vi "find splitting-fit lorentzian method.vi"(9 "E":dbl[][](graph)=array801x69[55269 elements], 10 "Y Scale":T2={"Offset"=-90000.0, "Multiplier"=2608.695652173913}, 11 "X Scale":T2={"Offset"=-0.09, "Multiplier"=8.5e-05}) -> (3 "XY Graph 4":cluster{dbl[], dbl[]}[](graph)=[{[-0.06773, -0.06773, -0.06824, -0.068325, -0.06841, -0.06841, -0.068325, -0.06806999999999999, -0.06773, -0.06773, -0.06773, -0.06773, -0.067645, -0.06738999999999999, -0.06722, -0.06705, -0.06670999999999999, -0.06637, -0.0662, -0.06602999999999999, -0.065775, -0.06552, -0.06534999999999999, -0.06517999999999999, -0.06509499999999999, -0.06484, -0.064585, -0.06416, -0.06841, -0.068665, -0.068835, -0.069005, -0.069005, -0.06909, -0.06909, -0.06917499999999999, -0.06925999999999999, -0.06917499999999999, -0.06917499999999999, -0.06909, -0.06909, -0.069005, -0.069005, -0.06909, -0.06909, -0.06892, -0.06874999999999999, -0.06874999999999999, -0.06874999999999999, -0.06773, -0.067475, -0.067645, -0.067645, -0.067645, -0.067645, -0.067475, -0.067475, -0.067475, -0.06738999999999999, -0.06756, -0.067475, -0.06738999999999999, -0.06738999999999999, -0.06738999999999999, -0.06722, -0.066965, -0.06670999999999999, -0.06645499999999999, -0.066115, -0.065945, -0.065605, -0.06534999999999999, -0.06517999999999999, -0.064925, -0.06466999999999999, -0.064245, -0.06398999999999999, -0.06381999999999999, -0.06390499999999999, -0.06433, -0.06398999999999999, -0.06398999999999999, -0.06841, -0.06858, -0.068835, -0.06892, -0.069005, -0.069005, -0.06909, -0.06909, -0.06909, -0.06917499999999999, -0.06925999999999999, -0.06925999999999999, -0.06942999999999999, -0.06934499999999999, -0.06934499999999999, -0.06942999999999999], [-1304.0, -1304.3478260869597, 1304.3478260869597, 3913.0434782608645, 6521.739130434784, 9130.434782608689, 11739.130434782608, 14347.826086956513, 16956.521739130432, 19565.21739130435, 22173.913043478256, 24782.608695652176, 27391.30434782608, 30000.0, 32608.695652173905, 35217.391304347824, 37826.08695652174, 40434.78260869565, 43043.47826086957, 45652.17391304349, 48260.86956521738, 50869.5652173913, 53478.260869565216, 56086.956521739135, 58695.652173913055, 61304.347826086945, 63913.043478260865, 66521.73913043478, 37826.08695652174, 40434.78260869565, 43043.47826086957, 45652.17391304349, 48260.86956521738, 50869.5652173913, 53478.260869565216, 56086.956521739135, 58695.652173913055, 61304.347826086945, 63913.043478260865, 66521.73913043478, 69130.4347826087, 71739.1304347826, 71739.1304347826, 74347.82608695651, 76956.52173913043, 79565.21739130435, 82173.91304347827, 84782.60869565216, 87391.30434782608, -1304.0, -3913.0434782608645, -9130.434782608703, -11739.130434782608, -14347.826086956527, -16956.521739130432, -19565.21739130435, -22173.913043478256, -24782.608695652176, -27391.304347826088, -30000.0, -32608.695652173912, -35217.391304347824, -37826.08695652174, -40434.782608695656, -43043.47826086957, -45652.17391304348, -48260.86956521739, -50869.565217391304, -53478.260869565216, -56086.95652173913, -58695.65217391304, -61304.34782608696, -63913.04347826087, -66521.73913043478, -69130.4347826087, -71739.13043478261, -74347.82608695653, -76956.52173913043, -79565.21739130435, -82173.91304347826, -84782.60869565218, -84782.60869565218, -50869.565217391304, -53478.260869565216, -56086.95652173913, -58695.65217391304, -61304.34782608696, -63913.04347826087, -66521.73913043478, -69130.4347826087, -71739.13043478261, -74347.82608695653, -76956.52173913043, -79565.21739130435, -82173.91304347826, -84782.60869565218, -84782.60869565218, -87391.30434782608]}])   [LabVIEW 2013]
uses:
  <vilib>/Utility/miscctls.llb/LVOffsetAndMultiplierTypeDef.ctl
  <vilib>/Analysis/baseanly.llb/Mean (DBL).vi
  <vilib>/Analysis/NI_AAL_SigProc.lvlib
  <vilib>/Analysis/NI_AALBase.lvlib
panel:
  out "size(s)":i32=1
  in  "Tab Control":T1(tab)
  out "E 2":dbl[][](graph)
  in  "OK Button":bool
  out "Peak Detector":cluster{"X":dbl, "Y":dbl}[](graph)=[{"X"=-0.07546499999999999, "Y"=-90000.0}, {"X"=-0.06398999999999999, "Y"=-90000.0}, {"X"=-0.07690999999999999, "Y"=-87391.30434782608}, {"X"=-0.06942999999999999, "Y"=-87391.30434782608}, {"X"=-0.076995, "Y"=-84782.60869565218}, {"X"=-0.06934499999999999, "Y"=-84782.60869565218}, {"X"=-0.06398999999999999, "Y"=-84782.60869565218}, {"X"=-0.077165, "Y"=-82173.91304347826}, {"X"=-0.06942999999999999, "Y"=-82173.91304347826}, {"X"=-0.06433, "Y"=-82173.91304347826}, {"X"=-0.07708, "Y"=-79565.21739130435}, {"X"=-0.06925999999999999, "Y"=-79565.21739130435}, {"X"=-0.06390499999999999, "Y"=-79565.21739130435}, {"X"=-0.07725, "Y"=-76956.52173913043}, {"X"=-0.06925999999999999, "Y"=-76956.52173913043}, {"X"=-0.06381999999999999, "Y"=-76956.52173913043}, {"X"=-0.07741999999999999, "Y"=-74347.82608695653}, {"X"=-0.06917499999999999, "Y"=-74347.82608695653}, {"X"=-0.06398999999999999, "Y"=-74347.82608695653}, {"X"=-0.07750499999999999, "Y"=-71739.13043478261}, {"X"=-0.06909, "Y"=-71739.13043478261}, {"X"=-0.064245, "Y"=-71739.13043478261}, {"X"=-0.06909, "Y"=-69130.4347826087}, {"X"=-0.06466999999999999, "Y"=-69130.4347826087}, {"X"=-0.06909, "Y"=-66521.73913043478}, {"X"=-0.064925, "Y"=-66521.73913043478}, {"X"=-0.069005, "Y"=-63913.04347826087}, {"X"=-0.06517999999999999, "Y"=-63913.04347826087}, {"X"=-0.069005, "Y"=-61304.34782608696}, {"X"=-0.06534999999999999, "Y"=-61304.34782608696}, {"X"=-0.06892, "Y"=-58695.65217391304}, {"X"=-0.065605, "Y"=-58695.65217391304}, {"X"=-0.068835, "Y"=-56086.95652173913}, {"X"=-0.065945, "Y"=-56086.95652173913}, {"X"=-0.06858, "Y"=-53478.260869565216}, {"X"=-0.066115, "Y"=-53478.260869565216}, {"X"=-0.06841, "Y"=-50869.565217391304}, {"X"=-0.06645499999999999, "Y"=-50869.565217391304}, {"X"=-0.06670999999999999, "Y"=-48260.86956521739}, {"X"=-0.066965, "Y"=-45652.17391304348}, {"X"=-0.06722, "Y"=-43043.47826086957}, {"X"=-0.06738999999999999, "Y"=-40434.782608695656}, {"X"=-0.06373499999999999, "Y"=-40434.782608695656}, {"X"=-0.06738999999999999, "Y"=-37826.08695652174}, {"X"=-0.06330999999999999, "Y"=-37826.08695652174}, {"X"=-0.06738999999999999, "Y"=-35217.391304347824}, {"X"=-0.06330999999999999, "Y"=-35217.391304347824}, {"X"=-0.067475, "Y"=-32608.695652173912}, {"X"=-0.06330999999999999, "Y"=-32608.695652173912}, {"X"=-0.06756, "Y"=-30000.0}, {"X"=-0.063055, "Y"=-30000.0}, {"X"=-0.06738999999999999, "Y"=-27391.304347826088}, {"X"=-0.067475, "Y"=-24782.608695652176}, {"X"=-0.067475, "Y"=-22173.913043478256}, {"X"=-0.067475, "Y"=-19565.21739130435}, {"X"=-0.067645, "Y"=-16956.521739130432}, {"X"=-0.067645, "Y"=-14347.826086956527}, {"X"=-0.067645, "Y"=-11739.130434782608}, {"X"=-0.067645, "Y"=-9130.434782608703}, {"X"=-0.067475, "Y"=-3913.0434782608645}, {"X"=-0.06773, "Y"=-1304.3478260869597}, {"X"=-0.06824, "Y"=1304.3478260869597}, {"X"=-0.068325, "Y"=3913.0434782608645}, {"X"=-0.06841, "Y"=6521.739130434784}, {"X"=-0.06841, "Y"=9130.434782608689}, {"X"=-0.068325, "Y"=11739.130434782608}, {"X"=-0.06806999999999999, "Y"=14347.826086956513}, {"X"=-0.06773, "Y"=16956.521739130432}, {"X"=-0.06773, "Y"=19565.21739130435}, {"X"=-0.06773, "Y"=22173.913043478256}, {"X"=-0.06365, "Y"=22173.913043478256}, {"X"=-0.06773, "Y"=24782.608695652176}, {"X"=-0.06381999999999999, "Y"=24782.608695652176}, {"X"=-0.067645, "Y"=27391.30434782608}, {"X"=-0.06390499999999999, "Y"=27391.30434782608}, {"X"=-0.06738999999999999, "Y"=30000.0}, {"X"=-0.06722, "Y"=32608.695652173905}, {"X"=-0.06705, "Y"=35217.391304347824}, {"X"=-0.06841, "Y"=37826.08695652174}, {"X"=-0.06670999999999999, "Y"=37826.08695652174}, {"X"=-0.068665, "Y"=40434.78260869565}, {"X"=-0.06637, "Y"=40434.78260869565}, {"X"=-0.068835, "Y"=43043.47826086957}, {"X"=-0.0662, "Y"=43043.47826086957}, {"X"=-0.069005, "Y"=45652.17391304349}, {"X"=-0.06602999999999999, "Y"=45652.17391304349}, {"X"=-0.069005, "Y"=48260.86956521738}, {"X"=-0.065775, "Y"=48260.86956521738}, {"X"=-0.06909, "Y"=50869.5652173913}, {"X"=-0.06552, "Y"=50869.5652173913}, {"X"=-0.06909, "Y"=53478.260869565216}, {"X"=-0.06534999999999999, "Y"=53478.260869565216}, {"X"=-0.06917499999999999, "Y"=56086.956521739135}, {"X"=-0.06517999999999999, "Y"=56086.956521739135}, {"X"=-0.06925999999999999, "Y"=58695.652173913055}, {"X"=-0.06509499999999999, "Y"=58695.652173913055}, {"X"=-0.06917499999999999, "Y"=61304.347826086945}, {"X"=-0.06484, "Y"=61304.347826086945}, {"X"=-0.07750499999999999, "Y"=63913.043478260865}, {"X"=-0.06917499999999999, "Y"=63913.043478260865}, {"X"=-0.064585, "Y"=63913.043478260865}, {"X"=-0.077335, "Y"=66521.73913043478}, {"X"=-0.06909, "Y"=66521.73913043478}, {"X"=-0.06416, "Y"=66521.73913043478}, {"X"=-0.07725, "Y"=69130.4347826087}, {"X"=-0.06909, "Y"=69130.4347826087}, {"X"=-0.06390499999999999, "Y"=69130.4347826087}, {"X"=-0.07708, "Y"=71739.1304347826}, {"X"=-0.069005, "Y"=71739.1304347826}, {"X"=-0.06365, "Y"=71739.1304347826}, {"X"=-0.076995, "Y"=74347.82608695651}, {"X"=-0.06909, "Y"=74347.82608695651}, {"X"=-0.06365, "Y"=74347.82608695651}, {"X"=-0.07690999999999999, "Y"=76956.52173913043}, {"X"=-0.06909, "Y"=76956.52173913043}, {"X"=-0.06390499999999999, "Y"=76956.52173913043}, {"X"=-0.07682499999999999, "Y"=79565.21739130435}, {"X"=-0.06892, "Y"=79565.21739130435}, {"X"=-0.063565, "Y"=79565.21739130435}, {"X"=-0.07674, "Y"=82173.91304347827}, {"X"=-0.06874999999999999, "Y"=82173.91304347827}, {"X"=-0.076485, "Y"=84782.60869565216}, {"X"=-0.06874999999999999, "Y"=84782.60869565216}, {"X"=-0.076315, "Y"=87391.30434782608}, {"X"=-0.06874999999999999, "Y"=87391.30434782608}]
  out "Loretzian":cluster{dbl, dbl}[](graph)
  in  "Lorentzian?":bool
  in  "threshold":dbl=0.13 format="%.2p"
  in  "width":i32=3 min=3
  in  "stop":bool
  in  "Match condition":cluster{"X in range":dbl, "Y in range":dbl}={"X in range"=0.0029999999999999983, "Y in range"=0.0}
  in  "Fit match condition":cluster{"X in range":dbl, "Y in range":dbl}={"X in range"=0.001, "Y in range"=3000.0}
  in  "Memory points":dbl=14.0 format="%#_13g"
  in  "Fit memory points":dbl=4.0
  in  "Mode":u16(ring) items=["Mode 0", "Mode 1"]
  out "Peak Detector 2":cluster{"X":dbl, "Y":dbl}[](graph)=[{"X"=-0.07546499999999999, "Y"=-90000.0}, {"X"=-0.06398999999999999, "Y"=-90000.0}, {"X"=-0.07690999999999999, "Y"=-87391.30434782608}, {"X"=-0.06942999999999999, "Y"=-87391.30434782608}, {"X"=-0.076995, "Y"=-84782.60869565218}, {"X"=-0.06934499999999999, "Y"=-84782.60869565218}, {"X"=-0.06398999999999999, "Y"=-84782.60869565218}, {"X"=-0.077165, "Y"=-82173.91304347826}, {"X"=-0.06942999999999999, "Y"=-82173.91304347826}, {"X"=-0.06433, "Y"=-82173.91304347826}, {"X"=-0.07708, "Y"=-79565.21739130435}, {"X"=-0.06925999999999999, "Y"=-79565.21739130435}, {"X"=-0.06390499999999999, "Y"=-79565.21739130435}, {"X"=-0.07725, "Y"=-76956.52173913043}, {"X"=-0.06925999999999999, "Y"=-76956.52173913043}, {"X"=-0.06381999999999999, "Y"=-76956.52173913043}, {"X"=-0.07741999999999999, "Y"=-74347.82608695653}, {"X"=-0.06917499999999999, "Y"=-74347.82608695653}, {"X"=-0.06398999999999999, "Y"=-74347.82608695653}, {"X"=-0.07750499999999999, "Y"=-71739.13043478261}, {"X"=-0.06909, "Y"=-71739.13043478261}, {"X"=-0.064245, "Y"=-71739.13043478261}, {"X"=-0.06909, "Y"=-69130.4347826087}, {"X"=-0.06466999999999999, "Y"=-69130.4347826087}, {"X"=-0.06909, "Y"=-66521.73913043478}, {"X"=-0.064925, "Y"=-66521.73913043478}, {"X"=-0.069005, "Y"=-63913.04347826087}, {"X"=-0.06517999999999999, "Y"=-63913.04347826087}, {"X"=-0.069005, "Y"=-61304.34782608696}, {"X"=-0.06534999999999999, "Y"=-61304.34782608696}, {"X"=-0.06892, "Y"=-58695.65217391304}, {"X"=-0.065605, "Y"=-58695.65217391304}, {"X"=-0.068835, "Y"=-56086.95652173913}, {"X"=-0.065945, "Y"=-56086.95652173913}, {"X"=-0.06858, "Y"=-53478.260869565216}, {"X"=-0.066115, "Y"=-53478.260869565216}, {"X"=-0.06841, "Y"=-50869.565217391304}, {"X"=-0.06645499999999999, "Y"=-50869.565217391304}, {"X"=-0.06670999999999999, "Y"=-48260.86956521739}, {"X"=-0.066965, "Y"=-45652.17391304348}, {"X"=-0.06722, "Y"=-43043.47826086957}, {"X"=-0.06738999999999999, "Y"=-40434.782608695656}, {"X"=-0.06373499999999999, "Y"=-40434.782608695656}, {"X"=-0.06738999999999999, "Y"=-37826.08695652174}, {"X"=-0.06330999999999999, "Y"=-37826.08695652174}, {"X"=-0.06738999999999999, "Y"=-35217.391304347824}, {"X"=-0.06330999999999999, "Y"=-35217.391304347824}, {"X"=-0.067475, "Y"=-32608.695652173912}, {"X"=-0.06330999999999999, "Y"=-32608.695652173912}, {"X"=-0.06756, "Y"=-30000.0}, {"X"=-0.063055, "Y"=-30000.0}, {"X"=-0.06738999999999999, "Y"=-27391.304347826088}, {"X"=-0.067475, "Y"=-24782.608695652176}, {"X"=-0.067475, "Y"=-22173.913043478256}, {"X"=-0.067475, "Y"=-19565.21739130435}, {"X"=-0.067645, "Y"=-16956.521739130432}, {"X"=-0.067645, "Y"=-14347.826086956527}, {"X"=-0.067645, "Y"=-11739.130434782608}, {"X"=-0.067645, "Y"=-9130.434782608703}, {"X"=-0.067475, "Y"=-3913.0434782608645}, {"X"=-0.06773, "Y"=-1304.3478260869597}, {"X"=-0.06824, "Y"=1304.3478260869597}, {"X"=-0.068325, "Y"=3913.0434782608645}, {"X"=-0.06841, "Y"=6521.739130434784}, {"X"=-0.06841, "Y"=9130.434782608689}, {"X"=-0.068325, "Y"=11739.130434782608}, {"X"=-0.06806999999999999, "Y"=14347.826086956513}, {"X"=-0.06773, "Y"=16956.521739130432}, {"X"=-0.06773, "Y"=19565.21739130435}, {"X"=-0.06773, "Y"=22173.913043478256}, {"X"=-0.06365, "Y"=22173.913043478256}, {"X"=-0.06773, "Y"=24782.608695652176}, {"X"=-0.06381999999999999, "Y"=24782.608695652176}, {"X"=-0.067645, "Y"=27391.30434782608}, {"X"=-0.06390499999999999, "Y"=27391.30434782608}, {"X"=-0.06738999999999999, "Y"=30000.0}, {"X"=-0.06722, "Y"=32608.695652173905}, {"X"=-0.06705, "Y"=35217.391304347824}, {"X"=-0.06841, "Y"=37826.08695652174}, {"X"=-0.06670999999999999, "Y"=37826.08695652174}, {"X"=-0.068665, "Y"=40434.78260869565}, {"X"=-0.06637, "Y"=40434.78260869565}, {"X"=-0.068835, "Y"=43043.47826086957}, {"X"=-0.0662, "Y"=43043.47826086957}, {"X"=-0.069005, "Y"=45652.17391304349}, {"X"=-0.06602999999999999, "Y"=45652.17391304349}, {"X"=-0.069005, "Y"=48260.86956521738}, {"X"=-0.065775, "Y"=48260.86956521738}, {"X"=-0.06909, "Y"=50869.5652173913}, {"X"=-0.06552, "Y"=50869.5652173913}, {"X"=-0.06909, "Y"=53478.260869565216}, {"X"=-0.06534999999999999, "Y"=53478.260869565216}, {"X"=-0.06917499999999999, "Y"=56086.956521739135}, {"X"=-0.06517999999999999, "Y"=56086.956521739135}, {"X"=-0.06925999999999999, "Y"=58695.652173913055}, {"X"=-0.06509499999999999, "Y"=58695.652173913055}, {"X"=-0.06917499999999999, "Y"=61304.347826086945}, {"X"=-0.06484, "Y"=61304.347826086945}, {"X"=-0.07750499999999999, "Y"=63913.043478260865}, {"X"=-0.06917499999999999, "Y"=63913.043478260865}, {"X"=-0.064585, "Y"=63913.043478260865}, {"X"=-0.077335, "Y"=66521.73913043478}, {"X"=-0.06909, "Y"=66521.73913043478}, {"X"=-0.06416, "Y"=66521.73913043478}, {"X"=-0.07725, "Y"=69130.4347826087}, {"X"=-0.06909, "Y"=69130.4347826087}, {"X"=-0.06390499999999999, "Y"=69130.4347826087}, {"X"=-0.07708, "Y"=71739.1304347826}, {"X"=-0.069005, "Y"=71739.1304347826}, {"X"=-0.06365, "Y"=71739.1304347826}, {"X"=-0.076995, "Y"=74347.82608695651}, {"X"=-0.06909, "Y"=74347.82608695651}, {"X"=-0.06365, "Y"=74347.82608695651}, {"X"=-0.07690999999999999, "Y"=76956.52173913043}, {"X"=-0.06909, "Y"=76956.52173913043}, {"X"=-0.06390499999999999, "Y"=76956.52173913043}, {"X"=-0.07682499999999999, "Y"=79565.21739130435}, {"X"=-0.06892, "Y"=79565.21739130435}, {"X"=-0.063565, "Y"=79565.21739130435}, {"X"=-0.07674, "Y"=82173.91304347827}, {"X"=-0.06874999999999999, "Y"=82173.91304347827}, {"X"=-0.076485, "Y"=84782.60869565216}, {"X"=-0.06874999999999999, "Y"=84782.60869565216}, {"X"=-0.076315, "Y"=87391.30434782608}, {"X"=-0.06874999999999999, "Y"=87391.30434782608}]
  out "Possitive splitting data":cluster{"Numeric":dbl, dbl}[][](array[cluster])=[[{"Numeric"=-0.06773, -1304.3478260869597}, {"Numeric"=0.0, 0.0}, {"Numeric"=0.0, 0.0}], [{"Numeric"=-0.06824, 1304.3478260869597}, {"Numeric"=0.0, 0.0}, {"Numeric"=0.0, 0.0}], [{"Numeric"=-0.068325, 3913.0434782608645}, {"Numeric"=0.0, 0.0}, {"Numeric"=0.0, 0.0}], [{"Numeric"=-0.06841, 6521.739130434784}, {"Numeric"=0.0, 0.0}, {"Numeric"=0.0, 0.0}], [{"Numeric"=-0.06841, 9130.434782608689}, {"Numeric"=0.0, 0.0}, {"Numeric"=0.0, 0.0}], [{"Numeric"=-0.068325, 11739.130434782608}, {"Numeric"=0.0, 0.0}, {"Numeric"=0.0, 0.0}], [{"Numeric"=-0.06806999999999999, 14347.826086956513}, {"Numeric"=0.0, 0.0}, {"Numeric"=0.0, 0.0}], [{"Numeric"=-0.06773, 16956.521739130432}, {"Numeric"=0.0, 0.0}, {"Numeric"=0.0, 0.0}], [{"Numeric"=-0.06773, 19565.21739130435}, {"Numeric"=0.0, 0.0}, {"Numeric"=0.0, 0.0}], [{"Numeric"=-0.06773, 22173.913043478256}, {"Numeric"=-0.06365, 22173.913043478256}, {"Numeric"=0.0, 0.0}], [{"Numeric"=-0.06773, 24782.608695652176}, {"Numeric"=-0.06381999999999999, 24782.608695652176}, {"Numeric"=0.0, 0.0}], [{"Numeric"=-0.067645, 27391.30434782608}, {"Numeric"=-0.06390499999999999, 27391.30434782608}, {"Numeric"=0.0, 0.0}], [{"Numeric"=-0.06738999999999999, 30000.0}, {"Numeric"=0.0, 0.0}, {"Numeric"=0.0, 0.0}], [{"Numeric"=-0.06722, 32608.695652173905}, {"Numeric"=0.0, 0.0}, {"Numeric"=0.0, 0.0}], [{"Numeric"=-0.06705, 35217.391304347824}, {"Numeric"=0.0, 0.0}, {"Numeric"=0.0, 0.0}], [{"Numeric"=-0.06841, 37826.08695652174}, {"Numeric"=-0.06670999999999999, 37826.08695652174}, {"Numeric"=0.0, 0.0}], [{"Numeric"=-0.068665, 40434.78260869565}, {"Numeric"=-0.06637, 40434.78260869565}, {"Numeric"=0.0, 0.0}], [{"Numeric"=-0.068835, 43043.47826086957}, {"Numeric"=-0.0662, 43043.47826086957}, {"Numeric"=0.0, 0.0}], [{"Numeric"=-0.069005, 45652.17391304349}, {"Numeric"=-0.06602999999999999, 45652.17391304349}, {"Numeric"=0.0, 0.0}], [{"Numeric"=-0.069005, 48260.86956521738}, {"Numeric"=-0.065775, 48260.86956521738}, {"Numeric"=0.0, 0.0}], [{"Numeric"=-0.06909, 50869.5652173913}, {"Numeric"=-0.06552, 50869.5652173913}, {"Numeric"=0.0, 0.0}], [{"Numeric"=-0.06909, 53478.260869565216}, {"Numeric"=-0.06534999999999999, 53478.260869565216}, {"Numeric"=0.0, 0.0}], [{"Numeric"=-0.06917499999999999, 56086.956521739135}, {"Numeric"=-0.06517999999999999, 56086.956521739135}, {"Numeric"=0.0, 0.0}], [{"Numeric"=-0.06925999999999999, 58695.652173913055}, {"Numeric"=-0.06509499999999999, 58695.652173913055}, {"Numeric"=0.0, 0.0}], [{"Numeric"=-0.06917499999999999, 61304.347826086945}, {"Numeric"=-0.06484, 61304.347826086945}, {"Numeric"=0.0, 0.0}], [{"Numeric"=-0.07750499999999999, 63913.043478260865}, {"Numeric"=-0.06917499999999999, 63913.043478260865}, {"Numeric"=-0.064585, 63913.043478260865}], [{"Numeric"=-0.077335, 66521.73913043478}, {"Numeric"=-0.06909, 66521.73913043478}, {"Numeric"=-0.06416, 66521.73913043478}], [{"Numeric"=-0.07725, 69130.4347826087}, {"Numeric"=-0.06909, 69130.4347826087}, {"Numeric"=-0.06390499999999999, 69130.4347826087}], [{"Numeric"=-0.07708, 71739.1304347826}, {"Numeric"=-0.069005, 71739.1304347826}, {"Numeric"=-0.06365, 71739.1304347826}], [{"Numeric"=-0.076995, 74347.82608695651}, {"Numeric"=-0.06909, 74347.82608695651}, {"Numeric"=-0.06365, 74347.82608695651}], [{"Numeric"=-0.07690999999999999, 76956.52173913043}, {"Numeric"=-0.06909, 76956.52173913043}, {"Numeric"=-0.06390499999999999, 76956.52173913043}], [{"Numeric"=-0.07682499999999999, 79565.21739130435}, {"Numeric"=-0.06892, 79565.21739130435}, {"Numeric"=-0.063565, 79565.21739130435}], [{"Numeric"=-0.07674, 82173.91304347827}, {"Numeric"=-0.06874999999999999, 82173.91304347827}, {"Numeric"=0.0, 0.0}], [{"Numeric"=-0.076485, 84782.60869565216}, {"Numeric"=-0.06874999999999999, 84782.60869565216}, {"Numeric"=0.0, 0.0}], [{"Numeric"=-0.076315, 87391.30434782608}, {"Numeric"=-0.06874999999999999, 87391.30434782608}, {"Numeric"=0.0, 0.0}]]
  out "Negative splitting data":cluster{"Numeric":dbl, dbl}[][](array[cluster])=[[{"Numeric"=-0.067475, -3913.0434782608645}, {"Numeric"=0.0, 0.0}, {"Numeric"=0.0, 0.0}], [{"Numeric"=0.0, 0.0}, {"Numeric"=0.0, 0.0}, {"Numeric"=0.0, 0.0}], [{"Numeric"=-0.067645, -9130.434782608703}, {"Numeric"=0.0, 0.0}, {"Numeric"=0.0, 0.0}], [{"Numeric"=-0.067645, -11739.130434782608}, {"Numeric"=0.0, 0.0}, {"Numeric"=0.0, 0.0}], [{"Numeric"=-0.067645, -14347.826086956527}, {"Numeric"=0.0, 0.0}, {"Numeric"=0.0, 0.0}], [{"Numeric"=-0.067645, -16956.521739130432}, {"Numeric"=0.0, 0.0}, {"Numeric"=0.0, 0.0}], [{"Numeric"=-0.067475, -19565.21739130435}, {"Numeric"=0.0, 0.0}, {"Numeric"=0.0, 0.0}], [{"Numeric"=-0.067475, -22173.913043478256}, {"Numeric"=0.0, 0.0}, {"Numeric"=0.0, 0.0}], [{"Numeric"=-0.067475, -24782.608695652176}, {"Numeric"=0.0, 0.0}, {"Numeric"=0.0, 0.0}], [{"Numeric"=-0.06738999999999999, -27391.304347826088}, {"Numeric"=0.0, 0.0}, {"Numeric"=0.0, 0.0}], [{"Numeric"=-0.06756, -30000.0}, {"Numeric"=-0.063055, -30000.0}, {"Numeric"=0.0, 0.0}], [{"Numeric"=-0.067475, -32608.695652173912}, {"Numeric"=-0.06330999999999999, -32608.695652173912}, {"Numeric"=0.0, 0.0}], [{"Numeric"=-0.06738999999999999, -35217.391304347824}, {"Numeric"=-0.06330999999999999, -35217.391304347824}, {"Numeric"=0.0, 0.0}], [{"Numeric"=-0.06738999999999999, -37826.08695652174}, {"Numeric"=-0.06330999999999999, -37826.08695652174}, {"Numeric"=0.0, 0.0}], [{"Numeric"=-0.06738999999999999, -40434.782608695656}, {"Numeric"=-0.06373499999999999, -40434.782608695656}, {"Numeric"=0.0, 0.0}], [{"Numeric"=-0.06722, -43043.47826086957}, {"Numeric"=0.0, 0.0}, {"Numeric"=0.0, 0.0}], [{"Numeric"=-0.066965, -45652.17391304348}, {"Numeric"=0.0, 0.0}, {"Numeric"=0.0, 0.0}], [{"Numeric"=-0.06670999999999999, -48260.86956521739}, {"Numeric"=0.0, 0.0}, {"Numeric"=0.0, 0.0}], [{"Numeric"=-0.06841, -50869.565217391304}, {"Numeric"=-0.06645499999999999, -50869.565217391304}, {"Numeric"=0.0, 0.0}], [{"Numeric"=-0.06858, -53478.260869565216}, {"Numeric"=-0.066115, -53478.260869565216}, {"Numeric"=0.0, 0.0}], [{"Numeric"=-0.068835, -56086.95652173913}, {"Numeric"=-0.065945, -56086.95652173913}, {"Numeric"=0.0, 0.0}], [{"Numeric"=-0.06892, -58695.65217391304}, {"Numeric"=-0.065605, -58695.65217391304}, {"Numeric"=0.0, 0.0}], [{"Numeric"=-0.069005, -61304.34782608696}, {"Numeric"=-0.06534999999999999, -61304.34782608696}, {"Numeric"=0.0, 0.0}], [{"Numeric"=-0.069005, -63913.04347826087}, {"Numeric"=-0.06517999999999999, -63913.04347826087}, {"Numeric"=0.0, 0.0}], [{"Numeric"=-0.06909, -66521.73913043478}, {"Numeric"=-0.064925, -66521.73913043478}, {"Numeric"=0.0, 0.0}], [{"Numeric"=-0.06909, -69130.4347826087}, {"Numeric"=-0.06466999999999999, -69130.4347826087}, {"Numeric"=0.0, 0.0}], [{"Numeric"=-0.07750499999999999, -71739.13043478261}, {"Numeric"=-0.06909, -71739.13043478261}, {"Numeric"=-0.064245, -71739.13043478261}], [{"Numeric"=-0.07741999999999999, -74347.82608695653}, {"Numeric"=-0.06917499999999999, -74347.82608695653}, {"Numeric"=-0.06398999999999999, -74347.82608695653}], [{"Numeric"=-0.07725, -76956.52173913043}, {"Numeric"=-0.06925999999999999, -76956.52173913043}, {"Numeric"=-0.06381999999999999, -76956.52173913043}], [{"Numeric"=-0.07708, -79565.21739130435}, {"Numeric"=-0.06925999999999999, -79565.21739130435}, {"Numeric"=-0.06390499999999999, -79565.21739130435}], [{"Numeric"=-0.077165, -82173.91304347826}, {"Numeric"=-0.06942999999999999, -82173.91304347826}, {"Numeric"=-0.06433, -82173.91304347826}], [{"Numeric"=-0.076995, -84782.60869565218}, {"Numeric"=-0.06934499999999999, -84782.60869565218}, {"Numeric"=-0.06398999999999999, -84782.60869565218}], [{"Numeric"=-0.07690999999999999, -87391.30434782608}, {"Numeric"=-0.06942999999999999, -87391.30434782608}, {"Numeric"=0.0, 0.0}], [{"Numeric"=-0.07546499999999999, -90000.0}, {"Numeric"=-0.06398999999999999, -90000.0}, {"Numeric"=0.0, 0.0}]]
  out "XY Graph 3":cluster{dbl[], dbl[]}[](graph)=[{[-0.06773, -0.067475, -0.067645, -0.067645, -0.067645, -0.067645, -0.067475, -0.067475, -0.067475, -0.06738999999999999, -0.06756, -0.067475, -0.06738999999999999, -0.06738999999999999, -0.06738999999999999, -0.06722, -0.066965, -0.06670999999999999], [-1304.0, -3913.0434782608645, -9130.434782608703, -11739.130434782608, -14347.826086956527, -16956.521739130432, -19565.21739130435, -22173.913043478256, -24782.608695652176, -27391.304347826088, -30000.0, -32608.695652173912, -35217.391304347824, -37826.08695652174, -40434.782608695656, -43043.47826086957, -45652.17391304348, -48260.86956521739]}, {[-0.06645499999999999, -0.066115, -0.065945, -0.065605, -0.06534999999999999, -0.06517999999999999, -0.064925, -0.06466999999999999, -0.064245, -0.06398999999999999, -0.06381999999999999, -0.06390499999999999, -0.06433, -0.06398999999999999, -0.06398999999999999], [-50869.565217391304, -53478.260869565216, -56086.95652173913, -58695.65217391304, -61304.34782608696, -63913.04347826087, -66521.73913043478, -69130.4347826087, -71739.13043478261, -74347.82608695653, -76956.52173913043, -79565.21739130435, -82173.91304347826, -84782.60869565218, -84782.60869565218]}, {[-0.06841, -0.06858, -0.068835, -0.06892, -0.069005, -0.069005, -0.06909, -0.06909, -0.06909, -0.06917499999999999, -0.06925999999999999, -0.06925999999999999, -0.06942999999999999, -0.06934499999999999, -0.06934499999999999, -0.06942999999999999], [-50869.565217391304, -53478.260869565216, -56086.95652173913, -58695.65217391304, -61304.34782608696, -63913.04347826087, -66521.73913043478, -69130.4347826087, -71739.13043478261, -74347.82608695653, -76956.52173913043, -79565.21739130435, -82173.91304347826, -84782.60869565218, -84782.60869565218, -87391.30434782608]}]
  out "XY Graph 2":cluster{dbl[], dbl[]}[](graph)=[{[-0.06773, -0.06773, -0.06824, -0.068325, -0.06841, -0.06841, -0.068325, -0.06806999999999999, -0.06773, -0.06773, -0.06773, -0.06773, -0.067645, -0.06738999999999999, -0.06722, -0.06705], [-1304.0, -1304.3478260869597, 1304.3478260869597, 3913.0434782608645, 6521.739130434784, 9130.434782608689, 11739.130434782608, 14347.826086956513, 16956.521739130432, 19565.21739130435, 22173.913043478256, 24782.608695652176, 27391.30434782608, 30000.0, 32608.695652173905, 35217.391304347824]}, {[-0.06670999999999999, -0.06637, -0.0662, -0.06602999999999999, -0.065775, -0.06552, -0.06534999999999999, -0.06517999999999999, -0.06509499999999999, -0.06484, -0.064585, -0.06416], [37826.08695652174, 40434.78260869565, 43043.47826086957, 45652.17391304349, 48260.86956521738, 50869.5652173913, 53478.260869565216, 56086.956521739135, 58695.652173913055, 61304.347826086945, 63913.043478260865, 66521.73913043478]}, {[-0.06841, -0.068665, -0.068835, -0.069005, -0.069005, -0.06909, -0.06909, -0.06917499999999999, -0.06925999999999999, -0.06917499999999999, -0.06917499999999999, -0.06909, -0.06909, -0.069005, -0.069005, -0.06909, -0.06909, -0.06892, -0.06874999999999999, -0.06874999999999999, -0.06874999999999999], [37826.08695652174, 40434.78260869565, 43043.47826086957, 45652.17391304349, 48260.86956521738, 50869.5652173913, 53478.260869565216, 56086.956521739135, 58695.652173913055, 61304.347826086945, 63913.043478260865, 66521.73913043478, 69130.4347826087, 71739.1304347826, 71739.1304347826, 74347.82608695651, 76956.52173913043, 79565.21739130435, 82173.91304347827, 84782.60869565216, 87391.30434782608]}]
  out "zero field seeds":cluster{"X":dbl, "Y":dbl}[](graph)=[{"X"=-0.06773, "Y"=-1304.3478260869597}]
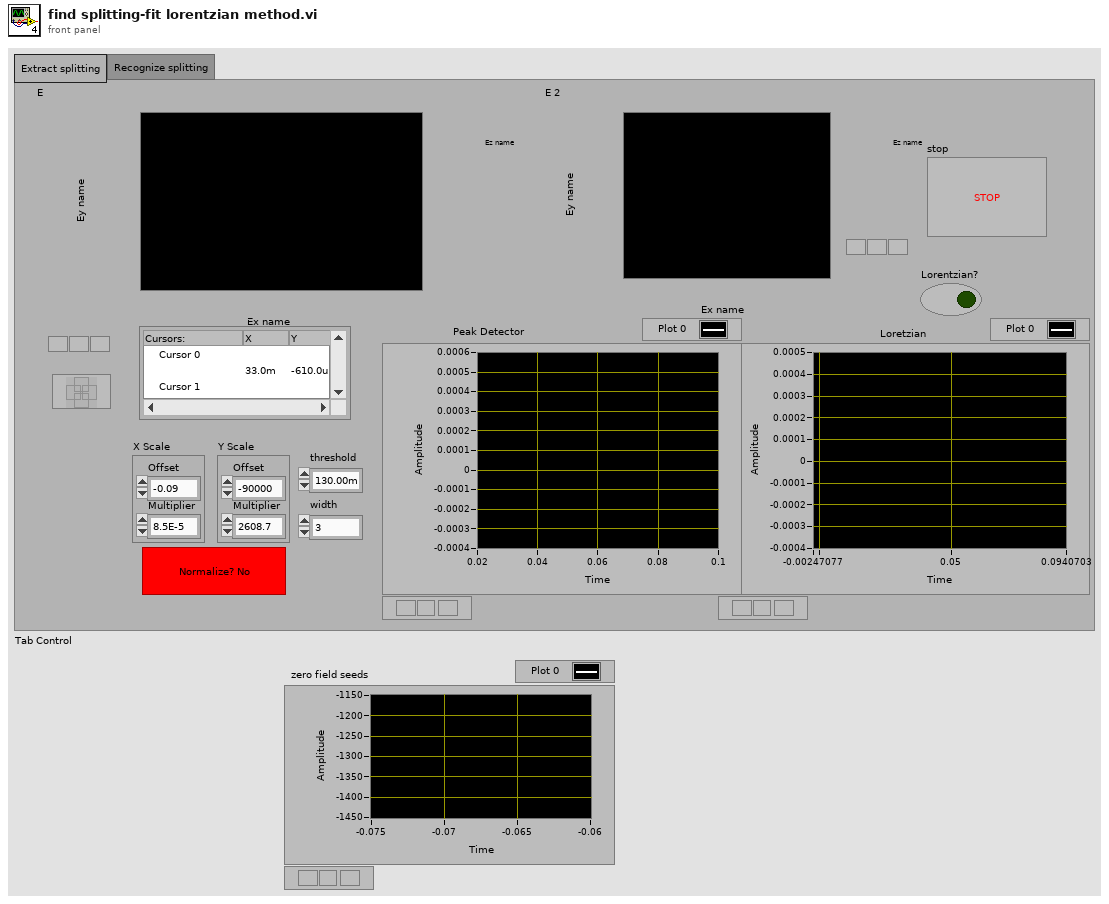
[diagram p1: front panel]
types:
  T1 = enum32{"Extract splitting", "Recognize splitting"}
  T2 = typedef "LVOffsetAndMultiplierTypeDef.ctl" = cluster{"Offset":dbl, "Multiplier":dbl}
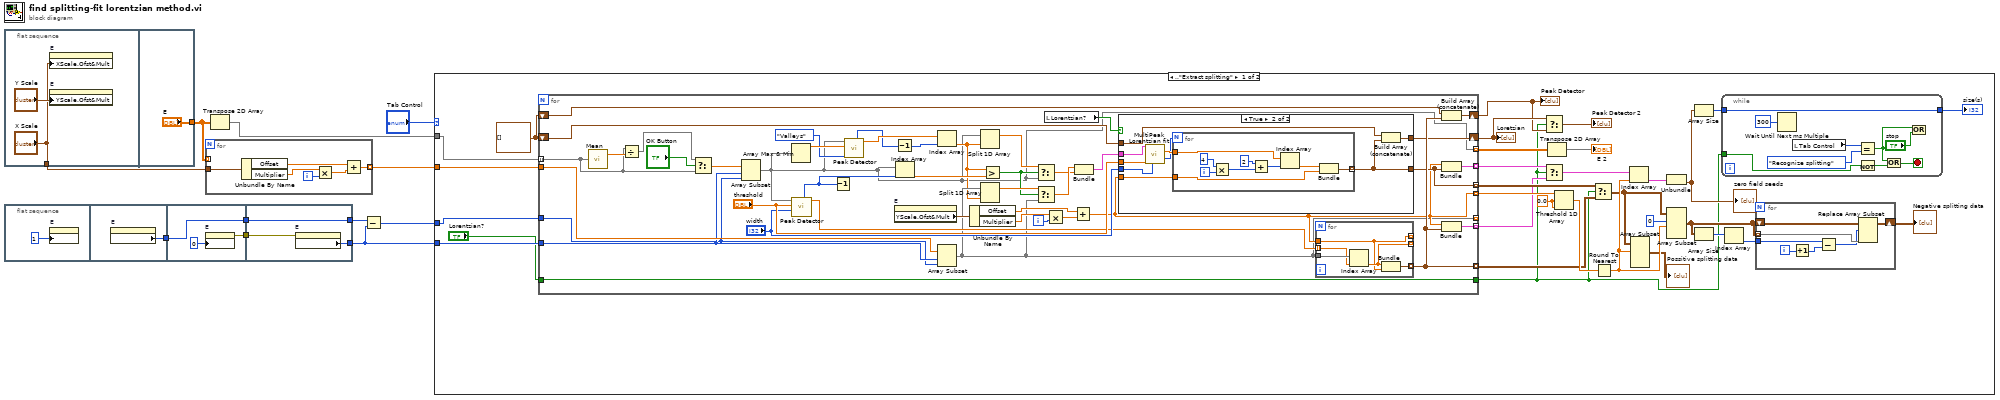
[diagram p0: block diagram]
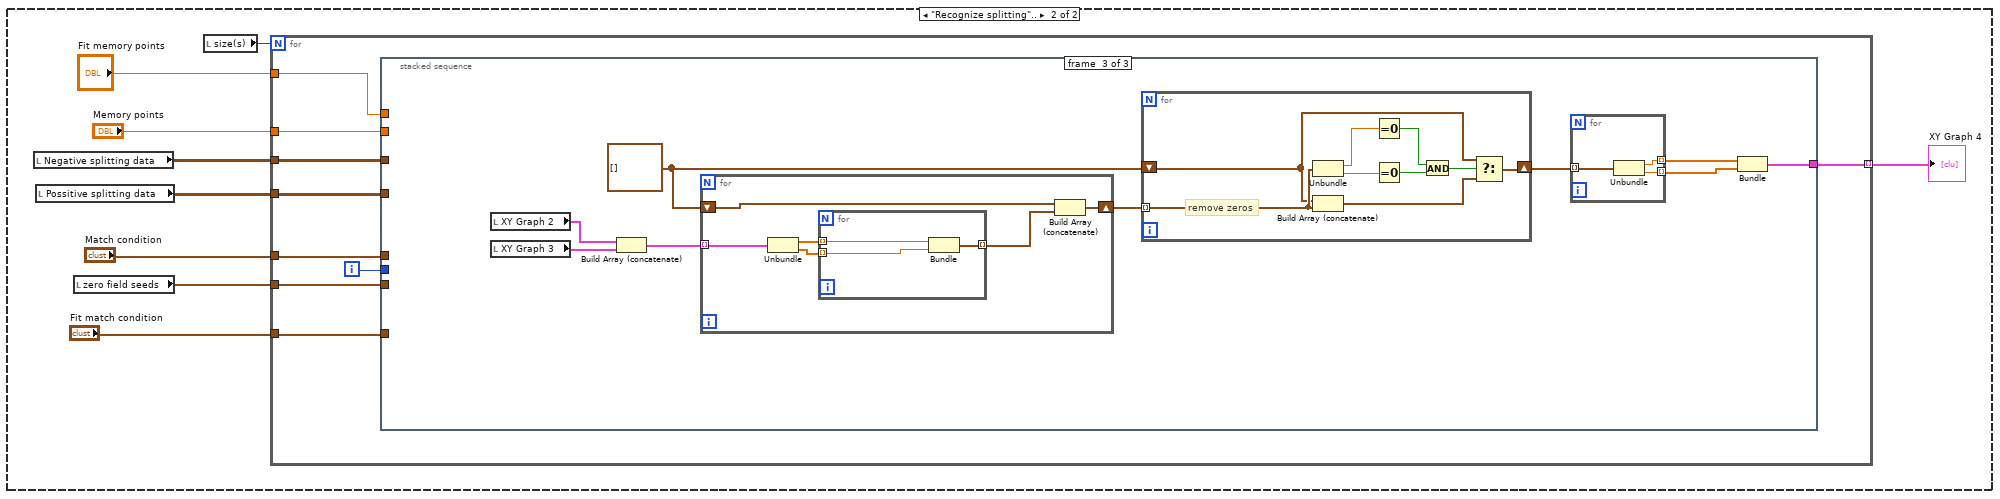
[diagram p3: hidden frame]
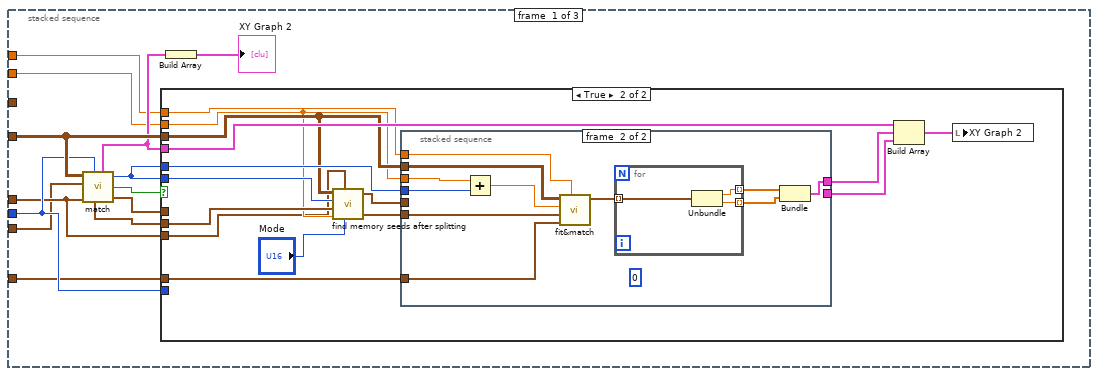
[diagram p4: hidden frame]
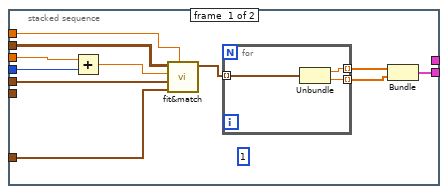
[diagram p6: hidden frame]
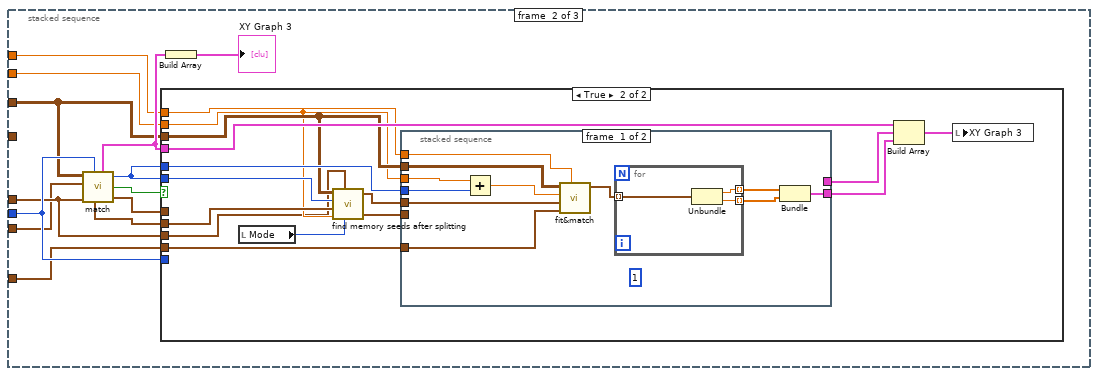
[diagram p7: hidden frame]
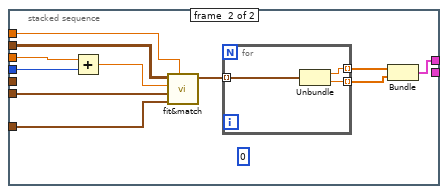
[diagram p9: hidden frame]
diagram:
  n1 = flat-sequence {
    tunnel: ["X Scale"] -> w9
    tunnel: ["E"] -> w10
    frame #0 {
      n2 = property on="E" class="IntGraph (strict)"("XScale.Ofst&Mult"="X Scale") -> ()  [unwired: 2 in, 2 out]
      n3 = property on="E" class="IntGraph (strict)"("YScale.Ofst&Mult"="Y Scale") -> ()  [unwired: 2 in, 2 out]
    }
    frame #1 {
    }
  }
  n4 = flat-sequence {
    tunnel: [w16] -> w5
    tunnel: [w18] -> w7
    tunnel: [w17] -> w6
    tunnel: w5 -> [w17]
    tunnel: w7 -> [w22]
    tunnel: [w21] -> w4
    tunnel: w6 -> [w21]
    tunnel: [w20] -> w2
    frame #0 {
      n5 = property on="E" class="IntGraph (strict)"("Active Cursor"=u32 1) -> ()  [unwired: 2 in, 2 out]
    }
    frame #1 {
      n6 = property on="E" class="IntGraph (strict)"() -> ("Cursor.Cursor Index"=w16:i32)  [unwired: 2 in, 2 out]
    }
    frame #2 {
      n7 = property on="E" class="IntGraph (strict)"("Active Cursor"=u32 0) -> (error out=w18:errorcluster)  [unwired: 2 in, 1 out]
    }
    frame #3 {
      n8 = property on="E" class="IntGraph (strict)"(error in=w22) -> ("Cursor.Cursor Index"=w20:i32)  [unwired: 1 in, 2 out]
    }
  }
  n9 = for {
    tunnel: w9 -> [w25]
    tunnel: w10 -> [_] mode=indexing
    tunnel: [w23] -> w8 mode=indexing
    i -> [w24]
    n10 = Unbundle By Name(w25) -> ("Offset"=w26:dbl, "Multiplier"=w27:dbl)
    n11 = Multiply(x=w27, y=w24) -> (x*y=w28:dbl)
    n12 = Add(x=w26, y=w28) -> (x+y=w23:dbl)
  }
  n13 = Transpose 2D Array(2D array=w10) -> (transposed array=w11:dbl[][])
  n14 = Subtract(x=w4, y=w2) -> (x-y=w3:i32)
  n15 = case shown="..\"Extract splitting\"" "Tab Control" {
    tunnel: w11 -> [w60 _]
    tunnel: w8 -> [w47 _]
    tunnel: w3 -> [w46 _]
    tunnel: w2 -> [w45 _]
    frame .."Extract splitting" {
      w59 = 0.0 ("threshold y")
      w43 = cluster{dbl, dbl}[] []
      n16 = for {
        tunnel: w60 -> [w108] mode=indexing
        tunnel: [w96] -> w57 mode=indexing
        tunnel: w47 -> [w106]
        shift-right: [w114] -> w34
        shift-left: w43 -> [w113]
        tunnel: [w112] -> w42 mode=indexing
        tunnel: [w111] -> w39 mode=indexing
        tunnel: w46 -> [w103]
        tunnel: w45 -> [w104]
        tunnel: [w78] -> w44 mode=indexing
        tunnel: [w83] -> _ mode=indexing
        shift-right: [w100] -> w35
        shift-left: w43 -> [w99]
        tunnel: [w97] -> w41 mode=indexing
        tunnel: [w94] -> w30
        tunnel: [w95] -> w37 mode=indexing
        tunnel: "Lorentzian?" -> [w94]
        i -> [w115]
        n17 = call-poly <vilib>:"Mean.vi"("X"=w108) -> ("mean"=w110:dbl)  [unwired: 1 out]
        n18 = Divide(x=w108, y=w110) -> (x/y=w109:dbl[])
        n19 = Select(t=w109, s="OK Button", f=w108) -> (s? t:f=w105:dbl[])
        n20 = Array Subset(array=w105, index=w104, length=w103) -> (w78:dbl[])
        n21 = Array Max & Min(array=w78) -> (max value=w91:dbl)  [unwired: 3 out]
        n22 = call <vilib>:"Peak Detector.vi"("width"="width", "threshold"="threshold", "X"=w78) -> ("Locations"=w92:dbl[], "# found"=w86:i32)  [unwired: 4 in, 3 out]
        n23 = Decrement(x=w86) -> ()  [unwired: 1 out]
        n24 = call <vilib>:"Peak Detector.vi"("peaks/valleys"=enum32{"Peaks", "Valleys"}."Valleys", "threshold"=w91, "X"=w78) -> ("Locations"=w89:dbl[], "# found"=w88:i32)  [unwired: 4 in, 3 out]
        n25 = property on="E" class="IntGraph (strict)"() -> ("YScale.Ofst&Mult"=w116:T2)  [unwired: 2 in, 2 out]
        n26 = Decrement(x=w88) -> (x-1=w87:i32)
        n27 = Index Array(array=w78, index=w86) -> (element=w85:dbl)
        n28 = Index Array(array=w89, index=w87) -> (element=w81:dbl)
        n29 = Array Subset(array=w106, index=w104, length=w103) -> (w83:dbl[])
        n30 = Unbundle By Name(w116) -> ("Offset"=w117:dbl, "Multiplier"=w118:dbl)
        n31 = Split 1D Array(array=w78, index=w81) -> (first subarray=w80:dbl[])  [unwired: 1 out]
        n32 = Split 1D Array(array=w83, index=w81) -> (first subarray=w84:dbl[])  [unwired: 1 out]
        n33 = Greater?(x=w81, y=w85) -> (0:w79:bool)
        n34 = Select(t=w80, s=w79, f=w78) -> (s? t:f=w77:dbl[])
        n35 = Select(t=w84, s=w79, f=w83) -> (s? t:f=w82:dbl[])
        n36 = local read "Lorentzian?"() -> (w93:bool)
        n37 = Multiply(x=w118, y=w115) -> (x*y=w119:dbl)
        n38 = Add(x=w117, y=w119) -> (x+y=w96:dbl)
        n39 = Bundle(w82, w77) -> (w98:cluster{dbl[], dbl[]})  [unwired: 1 in]
        n40 = case shown="True" w93 {
          tunnel: "threshold" -> [_ w129]
          tunnel: "width" -> [_ w128]
          tunnel: w96 -> [_ w125]
          tunnel: [w120 w124] -> w100
          tunnel: w99 -> [w120 w123]
          tunnel: w98 -> [_ w122]
          tunnel: [w120 w121] -> w97
          frame False {
          }
          frame True {
            n41 = call "MultiPeak Lorentzian fit.vi"("Data"=w122, "PD threshold"=w129, "PD width"=w128) -> ("best fit parameters"=w127:dbl[], "# of peaks"=w126:i32)  [unwired: 7 in, 4 out]
            n42 = for {
              N: w126 -> [_]
              tunnel: w127 -> [w138]
              tunnel: w125 -> [w134]
              tunnel: [w133] -> w121 mode=indexing
              i -> [w137]
              n43 = Multiply(x=4, y=w137) -> (x*y=w132:i32)
              n44 = Add(x=2, y=w132) -> (x+y=w130:i32)
              n45 = Index Array(array=w138, index=w130) -> (element=w135:dbl)
              n46 = Bundle("Numeric"=w135, w134) -> (w133:cluster{"Numeric":dbl, dbl})  [unwired: 1 in]
            }
            n47 = Build Array (concatenate)(w123, w121) -> (w124:cluster{"Numeric":dbl, dbl}[])
          }
        }
        n48 = for {
          tunnel: w83 -> [w143]
          tunnel: w92 -> [w142] mode=indexing
          tunnel: w96 -> [w140]
          tunnel: [w140] -> _ mode=indexing
          tunnel: [w141] -> _ mode=indexing
          tunnel: [w139] -> w112 mode=indexing
          n49 = Index Array(array=w143, index=w142) -> (element=w141:dbl)
          n50 = Bundle(w141, w140) -> (w139:cluster{dbl, dbl})  [unwired: 1 in]
        }
        n51 = Build Array (concatenate)(w113, w112) -> (w114:cluster{dbl, dbl}[])
        n52 = Bundle(w96, w97) -> (w95:cluster{dbl, cluster{"Numeric":dbl, dbl}[]})  [unwired: 1 in]
        n53 = Bundle(w96, w112) -> (w111:cluster{dbl, cluster{dbl, dbl}[]})  [unwired: 1 in]
      }
      "Peak Detector" <- w34
      "Loretzian" <- w35
      n54 = Select(t=w35, s=w30, f=w34) -> (s? t:f=→"Peak Detector 2":cluster{dbl, dbl}[])
      n55 = Select(t=w37, s=w30, f=w39) -> (s? t:f=w38:cluster{dbl, cluster{"Numeric":dbl, dbl}[]}[])
      n56 = Transpose 2D Array(2D array=w44) -> (transposed array=→"E 2":dbl[][])
      n57 = Threshold 1D Array(1:w59, 2:w59, 3:w57) -> (0:w58:dbl)
      n58 = Select(t=w41, s=w30, f=w42) -> (s? t:f=w40:cluster{"Numeric":dbl, dbl}[][])
      n59 = Round To Nearest(number=w58) -> (nearest integer value=w54:dbl)
      n60 = Index Array(array=w38, index=w54) -> (element=w56:cluster{dbl, cluster{"Numeric":dbl, dbl}[]})
      n61 = Array Subset(array=w40, index (row)=w54) -> (→"Possitive splitting data":cluster{"Numeric":dbl, dbl}[][])  [unwired: 3 in]
      n62 = Unbundle(w56) -> (w49:cluster{"Numeric":dbl, dbl}[])  [unwired: 1 out]
      "zero field seeds" <- w49
      n63 = Array Subset(array=w40, index (row)=0 ("index"), length (row)=w54) -> (w51:cluster{"Numeric":dbl, dbl}[][])  [unwired: 2 in]
      n64 = Array Size(array=w49) -> (size(s)=w32:i32)
      n65 = Array Size(array=w51) -> (size(s)=w53:i32[])
      n66 = while {
        tunnel: w32 -> [w69]
        tunnel: [w69] -> w31
        tunnel: w30 -> [w64]
        stop <- w63 stop-if-true
        n67 = Wait Until Next ms Multiple(millisecond multiple=u32 300) -> ()  [unwired: 1 out]
        n68 = local read "Tab Control"() -> (w68:T1)
        n69 = Equal?(x=w68, y=T1."Recognize splitting") -> (x = y?=w65:bool)
        n70 = Not(x=w64) -> (.not. x?=w62:bool)
        n71 = Or(x=w65, y=w62) -> (x .or. y?=w63:bool)
        n72 = Or(x=w65, y="stop") -> ()  [unwired: 1 out]
      }
      "size(s)" <- w31
      n73 = Index Array(array=w53) -> (element=w52:i32)  [unwired: 1 in]
      n74 = for {
        tunnel: w51 -> [w76] mode=indexing
        tunnel: w52 -> [w74]
        shift-right: [w70] -> w50
        shift-left: w51 -> [w71]
        i -> [w75]
        n75 = Increment(x=w75) -> (x+1=w73:i32)
        n76 = Subtract(x=w74, y=w73) -> (x-y=w72:i32)
        n77 = Replace Array Subset(array=w71, new element=w76, index (row)=w72) -> (w70:cluster{"Numeric":dbl, dbl}[][])  [unwired: 1 in]
      }
      "Negative splitting data" <- w50
    }
    frame "Recognize splitting".. {
      n78 = local read "Negative splitting data"() -> (w148:cluster{"Numeric":dbl, dbl}[][])
      n79 = local read "Possitive splitting data"() -> (w147:cluster{"Numeric":dbl, dbl}[][])
      n80 = local read "zero field seeds"() -> (w146:cluster{"X":dbl, "Y":dbl}[])
      n81 = local read "size(s)"() -> (w145:i32)
      n82 = for {
        N: w145 -> [_]
        tunnel: w147 -> [w161]
        tunnel: "Match condition" -> [w160]
        tunnel: w146 -> [w159]
        tunnel: "Memory points" -> [w158]
        tunnel: "Fit match condition" -> [w157]
        tunnel: w148 -> [w156]
        tunnel: [w154] -> w144 mode=indexing
        tunnel: "Fit memory points" -> [w153]
        i -> [w155]
        n83 = stacked-sequence {
          tunnel: w161 -> [w172 _ _]
          tunnel: w155 -> [w171 w228 _]
          tunnel: w160 -> [w170 w227 _]
          tunnel: w159 -> [w167 w225 _]
          tunnel: w158 -> [w166 w224 _]
          tunnel: w157 -> [w164 w222 _]
          tunnel: w156 -> [_ w218 _]
          tunnel: [_ _ w277] -> w154
          tunnel: w153 -> [w163 w221 _]
          frame #0 {
            n84 = call "match.vi"("Match condition"=w170, "seed point index"=w171, "Seed array"=w167, "splitting data"=w172) -> ("New seeds"=w173:cluster{dbl, dbl}[], "Split occurs?"=w174:bool, "last data index"=w162:i32, "extracted splitting"=w169:cluster{dbl[], dbl[]}, "last point"=w165:cluster{dbl, dbl})  [unwired: 2 in]
            n85 = case shown="True" w174 {
              tunnel: w173 -> [_ _]
              tunnel: w172 -> [_ w181]
              tunnel: w171 -> [_ _]
              tunnel: w170 -> [_ w177]
              tunnel: w162 -> [_ w189]
              tunnel: w169 -> [_ w188]
              tunnel: w166 -> [_ w178]
              tunnel: w165 -> [_ w179]
              tunnel: w164 -> [_ w184]
              tunnel: w163 -> [_ w183]
              tunnel: w162 -> [_ w180]
              frame False {
              }
              frame True {
                n86 = call "find memory seeds after splitting.vi"("Mode"="Mode", "Memory points"=w178, "last point"=w179, "Match condition"=w177, "last data index"=w180, "splitting data"=w181) -> ("branch R seeds"=w175:cluster{dbl, dbl}[], "branch L seeds"=w182:cluster{dbl, dbl}[])  [unwired: 3 in]
                n87 = stacked-sequence {
                  tunnel: w181 -> [w200 w214]
                  tunnel: w189 -> [w193 w208]
                  tunnel: w184 -> [w198 w212]
                  tunnel: [_ w206] -> w187
                  tunnel: [w194 _] -> w186
                  tunnel: w178 -> [w192 w207]
                  tunnel: w183 -> [w191 w205]
                  tunnel: w182 -> [w190 _]
                  tunnel: w175 -> [_ w204]
                  frame #0 {
                    (unwired) 1 ("which splitting branch?")
                    n88 = Add(x=w192, y=w193) -> (x+y=w199:dbl)
                    n89 = call "fit&match.vi"("Fit memory points"=w191, "Match condition"=w198, "Splitting brach seeds"=w190, "start Index"=w199, "splitting data"=w200) -> ("Seed array 3"=w197:cluster{dbl, dbl}[])  [unwired: 3 in]
                    n90 = for {
                      tunnel: w197 -> [w203] mode=indexing
                      tunnel: [w202] -> w196 mode=indexing
                      tunnel: [w201] -> w195 mode=indexing
                      n91 = Unbundle(w203) -> (w202:dbl, w201:dbl)
                    }
                    n92 = Bundle(w196, w195) -> (w194:cluster{dbl[], dbl[]})  [unwired: 1 in]
                  }
                  frame #1 {
                    (unwired) 0 ("which splitting branch?")
                    n93 = Add(x=w207, y=w208) -> (x+y=w213:dbl)
                    n94 = call "fit&match.vi"("Fit memory points"=w205, "Match condition"=w212, "Splitting brach seeds"=w204, "start Index"=w213, "splitting data"=w214) -> ("Seed array 3"=w211:cluster{dbl, dbl}[])  [unwired: 3 in]
                    n95 = for {
                      tunnel: w211 -> [w217] mode=indexing
                      tunnel: [w216] -> w210 mode=indexing
                      tunnel: [w215] -> w209 mode=indexing
                      n96 = Unbundle(w217) -> (w216:dbl, w215:dbl)
                    }
                    n97 = Bundle(w210, w209) -> (w206:cluster{dbl[], dbl[]})  [unwired: 1 in]
                  }
                }
                n98 = Build Array(w188, w187, w186) -> (w185:cluster{dbl[], dbl[]}[])
                n99 = local write "XY Graph 2"(w185) -> ()
              }
            }
            n100 = Build Array(w169) -> (→"XY Graph 2":cluster{dbl[], dbl[]}[])
          }
          frame #1 {
            n101 = call "match.vi"("Match condition"=w227, "seed point index"=w228, "Seed array"=w225, "splitting data"=w218) -> ("New seeds"=w229:cluster{dbl, dbl}[], "Split occurs?"=w230:bool, "last data index"=w220:i32, "extracted splitting"=w226:cluster{dbl[], dbl[]}, "last point"=w223:cluster{dbl, dbl})  [unwired: 2 in]
            n102 = case shown="True" w230 {
              tunnel: w229 -> [_ _]
              tunnel: w218 -> [_ w238]
              tunnel: w228 -> [_ _]
              tunnel: w227 -> [_ w234]
              tunnel: w220 -> [_ w245]
              tunnel: w226 -> [_ w244]
              tunnel: w224 -> [_ w235]
              tunnel: w223 -> [_ w236]
              tunnel: w222 -> [_ w241]
              tunnel: w221 -> [_ w240]
              tunnel: w220 -> [_ w237]
              frame False {
              }
              frame True {
                n103 = local read "Mode"() -> (w231:u16)
                n104 = call "find memory seeds after splitting.vi"("Mode"=w231, "Memory points"=w235, "last point"=w236, "Match condition"=w234, "last data index"=w237, "splitting data"=w238) -> ("branch R seeds"=w233:cluster{dbl, dbl}[], "branch L seeds"=w239:cluster{dbl, dbl}[])  [unwired: 3 in]
                n105 = stacked-sequence {
                  tunnel: w238 -> [w256 w270]
                  tunnel: w245 -> [w249 w264]
                  tunnel: w241 -> [w254 w268]
                  tunnel: [_ w262] -> w243
                  tunnel: [w250 _] -> w242
                  tunnel: w235 -> [w248 w263]
                  tunnel: w240 -> [w247 w261]
                  tunnel: w239 -> [w246 _]
                  tunnel: w233 -> [_ w260]
                  frame #0 {
                    (unwired) 1 ("which splitting branch?")
                    n106 = Add(x=w248, y=w249) -> (x+y=w255:dbl)
                    n107 = call "fit&match.vi"("Fit memory points"=w247, "Match condition"=w254, "Splitting brach seeds"=w246, "start Index"=w255, "splitting data"=w256) -> ("Seed array 3"=w253:cluster{dbl, dbl}[])  [unwired: 3 in]
                    n108 = for {
                      tunnel: w253 -> [w259] mode=indexing
                      tunnel: [w258] -> w252 mode=indexing
                      tunnel: [w257] -> w251 mode=indexing
                      n109 = Unbundle(w259) -> (w258:dbl, w257:dbl)
                    }
                    n110 = Bundle(w252, w251) -> (w250:cluster{dbl[], dbl[]})  [unwired: 1 in]
                  }
                  frame #1 {
                    (unwired) 0 ("which splitting branch?")
                    n111 = Add(x=w263, y=w264) -> (x+y=w269:dbl)
                    n112 = call "fit&match.vi"("Fit memory points"=w261, "Match condition"=w268, "Splitting brach seeds"=w260, "start Index"=w269, "splitting data"=w270) -> ("Seed array 3"=w267:cluster{dbl, dbl}[])  [unwired: 3 in]
                    n113 = for {
                      tunnel: w267 -> [w273] mode=indexing
                      tunnel: [w272] -> w266 mode=indexing
                      tunnel: [w271] -> w265 mode=indexing
                      n114 = Unbundle(w273) -> (w272:dbl, w271:dbl)
                    }
                    n115 = Bundle(w266, w265) -> (w262:cluster{dbl[], dbl[]})  [unwired: 1 in]
                  }
                }
                n116 = Build Array(w244, w243, w242) -> (w232:cluster{dbl[], dbl[]}[])
                n117 = local write "XY Graph 3"(w232) -> ()
              }
            }
            n118 = Build Array(w226) -> (→"XY Graph 3":cluster{dbl[], dbl[]}[])
          }
          frame #2 {
            w275 = cluster{dbl, dbl}[] []
            n119 = local read "XY Graph 2"() -> (w282:cluster{dbl[], dbl[]}[])
            n120 = local read "XY Graph 3"() -> (w281:cluster{dbl[], dbl[]}[])
            n121 = Build Array (concatenate)(w282, w281) -> (w280:cluster{dbl[], dbl[]}[])
            n122 = for {
              tunnel: w280 -> [w300] mode=indexing
              shift-right: [w296] -> w276
              shift-left: w275 -> [w295]
              n123 = Unbundle(w300) -> (w299:dbl[], w298:dbl[])
              n124 = for {
                tunnel: w299 -> [w303] mode=indexing
                tunnel: w298 -> [w302] mode=indexing
                tunnel: [w301] -> w297 mode=indexing
                n125 = Bundle(w303, w302) -> (w301:cluster{dbl, dbl})  [unwired: 1 in]
              }
              n126 = Build Array (concatenate)(w295, w297) -> (w296:cluster{dbl, dbl}[])
            }
            n127 = for {
              tunnel: w276 -> [w286] mode=indexing
              shift-right: [w284] -> w274
              shift-left: w275 -> [w283]
              # "remove zeros"
              n128 = Unbundle(w286) -> (w291:dbl, w290:dbl)
              n129 = Build Array (concatenate)(w283, w286) -> (w285:cluster{dbl, dbl}[])
              n130 = Equal To 0?(x=w291) -> (x = 0?=w289:bool)
              n131 = Equal To 0?(x=w290) -> (x = 0?=w288:bool)
              n132 = And(x=w289, y=w288) -> (x .and. y?=w287:bool)
              n133 = Select(t=w283, s=w287, f=w285) -> (s? t:f=w284:cluster{dbl, dbl}[])
            }
            n134 = for {
              tunnel: w274 -> [w294] mode=indexing
              tunnel: [w293] -> w279 mode=indexing
              tunnel: [w292] -> w278 mode=indexing
              n135 = Unbundle(w294) -> (w293:dbl, w292:dbl)
            }
            n136 = Bundle(w279, w278) -> (w277:cluster{dbl[], dbl[]})  [unwired: 1 in]
          }
        }
      }
      "XY Graph 4" <- w144
    }
  }
